vi "FlatToRichni_bus_monitor_api_Frame.vi"(5 "OutputClusterType":T1, 11 "InputCluster":T2) -> (3 "OutputCluster":T1)   [LabVIEW 2025, in "bus_monitor_server.lvlib"]
uses:
  bus_monitor_server.lvlib
  ni_bus_monitor_api_Frame_Flat.ctl
  ni_bus_monitor_api_Frame.ctl
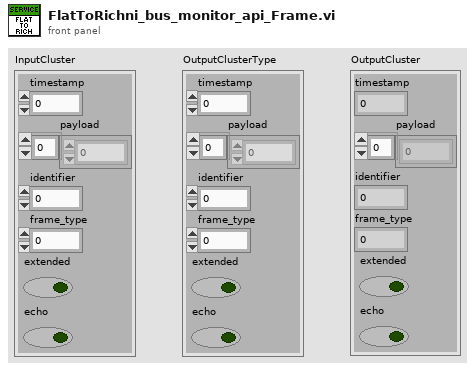
[diagram p1: front panel]
types:
  T1 = typedef "bus_monitor_server.lvlib/ni_bus_monitor_api_Frame.ctl" = cluster{"timestamp":dbl, "payload":u8[], "identifier":u32, "frame_type":u32, "extended":bool, "echo":bool}
  T2 = typedef "bus_monitor_server.lvlib/ni_bus_monitor_api_Frame_Flat.ctl" = cluster{"timestamp":dbl, "payload":u8[], "identifier":u32, "frame_type":u32, "extended":bool, "echo":bool}
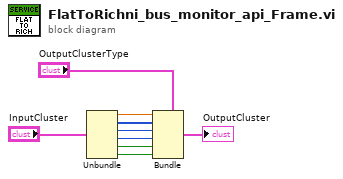
[diagram p0: block diagram]
diagram:
  n1 = Unbundle "Unbundle"("InputCluster") -> ("timestamp"=w6:dbl, "payload"=w5:u8[], "identifier"=w4:u32, "frame_type"=w3:u32, "extended"=w2:bool, "echo"=w1:bool)
  n2 = Bundle "Bundle"(cluster="OutputClusterType", "timestamp"=w6, "payload"=w5, "identifier"=w4, "frame_type"=w3, "extended"=w2, "echo"=w1) -> (→"OutputCluster":T1)
